vi "SaveAutoFile.vi"(9 "Ascript Data":string[](array[string]), 10 "Filename":string="RobotStateLog_", 11 "Base path":path) -> (3 "Filepath":path)   [LabVIEW 2016]
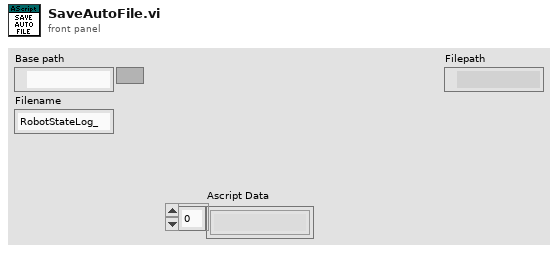
[diagram p1: front panel]
types:
  T1 = enum16{"open", "replace", "create", "open or create", "replace or create", "replace or create with confirmation"}
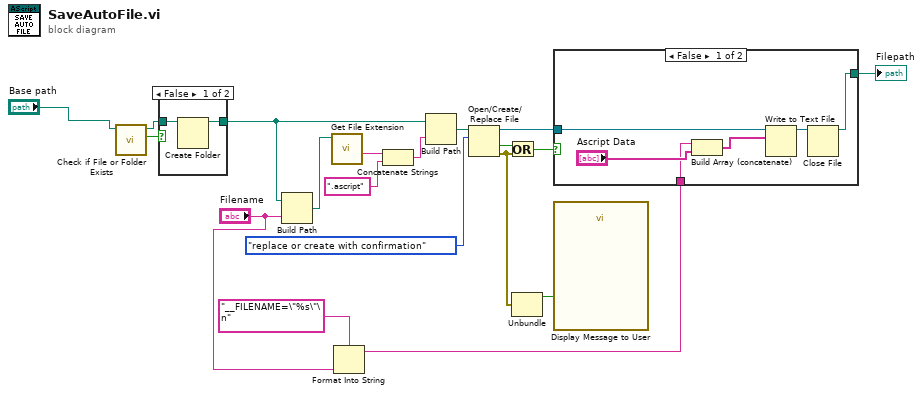
[diagram p0: block diagram]
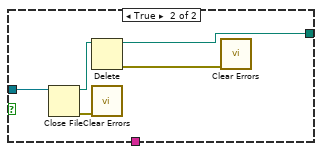
[diagram p2: hidden frame]
diagram:
  n1 = call <vilib>:"Check if File or Folder Exists.vi"("path"="Base path") -> ("file or folder exists?"=w19:bool, "dup path"=w18:path)  [unwired: 8 in, 1 out]
  n2 = case shown="False" w19 {
    tunnel: [w20 w22] -> w17
    tunnel: w18 -> [w21 w22]
    frame False {
      n3 = Create Folder(path (use dialog)=w21) -> (created path=w20:path)  [unwired: 2 in, 2 out]
    }
    frame True {
    }
  }
  n4 = Build Path(base path=w17, name or relative path="Filename") -> (appended path=w14:path)
  n5 = call <vilib>:"Get File Extension.vi"("file"=w14) -> ("filename without extension"=w13:string)  [unwired: 6 in, 4 out]
  n6 = Format Into String(format string="__FILENAME=\"%s\"\n" ("Filename"), "Filename") -> (resulting string=w2:string)  [unwired: 2 in, 1 out]
  n7 = Concatenate Strings(w13, ".ascript" ("string")) -> (w11:string)
  n8 = Build Path(base path=w17, name or relative path=w11) -> (appended path=w10:path)
  n9 = Open/Create/Replace File(file path (use dialog)=w10, operation (0:open)=T1."replace or create with confirmation") -> (refnum out=w16:refnum<file>, cancelled=w8:bool, error out=w5:errorcluster)  [unwired: 4 in]
  n10 = Or(x=w8, y=w5) -> (x .or. y?=w7:bool)
  n11 = Unbundle(w5) -> ("status"=w6:bool)  [unwired: 2 out]
  n12 = case shown="False" w7 {
    tunnel: w16 -> [w28 w33]
    tunnel: [w27 w31] -> w15
    tunnel: w2 -> [w24 _]
    frame False {
      n13 = Build Array (concatenate)(w24, "Ascript Data") -> (w23:string[])
      n14 = Write to Text File(file (use dialog)=w28, text=w23) -> (refnum out=w26:refnum<file>)  [unwired: 2 in, 2 out]
      n15 = Close File(refnum=w26) -> (path=w27:path)  [unwired: 1 in, 1 out]
    }
    frame True {
      n16 = Close File(refnum=w33) -> (path=w32:path, error out=w30:errorcluster)  [unwired: 1 in]
      n17 = Delete(path (use dialog)=w32) -> (deleted path=w31:path, error out=w29:errorcluster)  [unwired: 4 in, 1 out]
      n18 = call <vilib>:"Clear Errors.vi"("error in (no error)"=w30) -> ()  [unwired: 5 in, 2 out]
      n19 = call <vilib>:"Clear Errors.vi"("error in (no error)"=w29) -> ()  [unwired: 5 in, 2 out]
    }
  }
  "Filepath" <- w15
  n20 = call "Display Message to User"("Enable"=w6) -> ()  [unwired: 9 in, 2 out]
